vi "Calc_Vres.vi"(10 "S_Data in":dbl, 11 "P_Data in":dbl) -> (1 "Vres_FD":i32, 2 "Vres":dbl, 3 "Angle out":dbl)   [LabVIEW 2020]
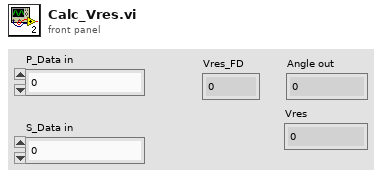
[diagram p1: front panel]
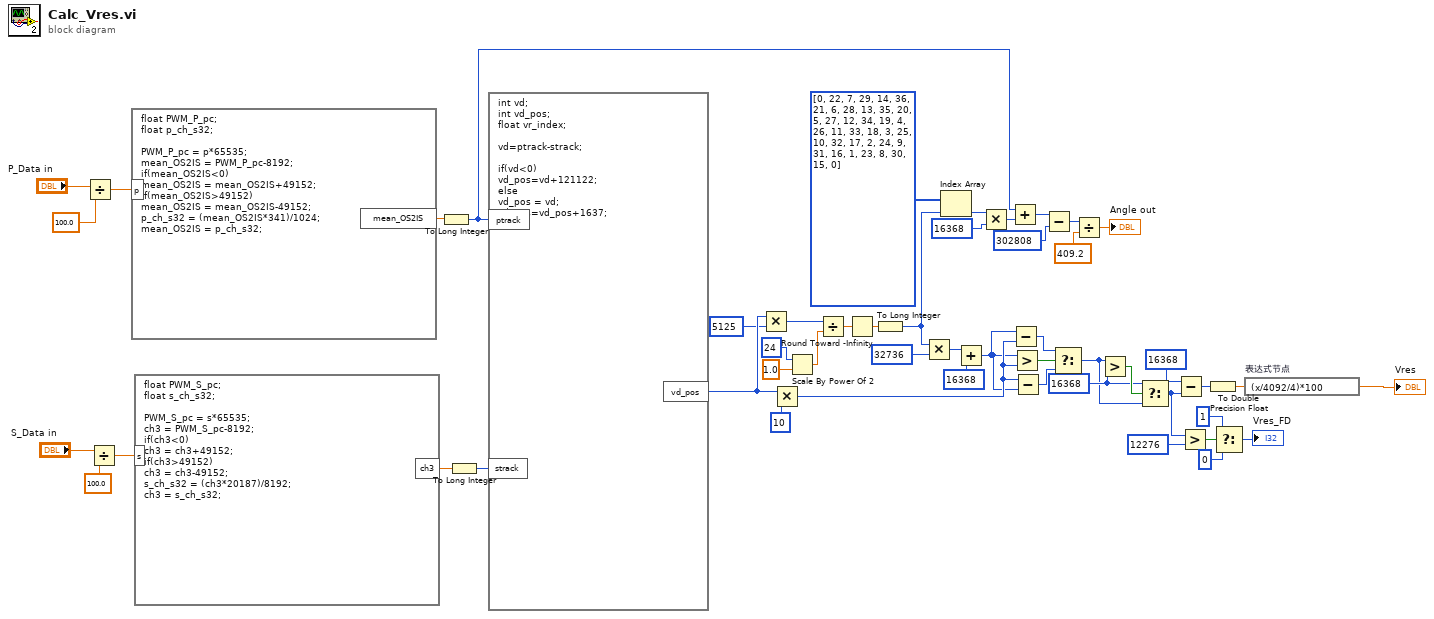
[diagram p0: block diagram]
diagram:
  w25 = 16368 ("y")
  n1 = Divide(x="P_Data in", y=100.0) -> (x/y=w12:dbl)
  n2 = Divide(x="S_Data in", y=100.0) -> (x/y=w10:dbl)
  n3 = formula code="float PWM_P_pc;\nfloat p_ch_s32;\n\nPWM_P_pc = p*65535;\nmean_OS2IS = PWM_P_pc-8192;\nif(mean_OS2IS<0)\nmean_OS2IS = mean_OS2IS+49152;\nif(mean_OS2IS>49152)\nmean_OS2IS = mean_OS2IS-49152;\np_ch_s32 = (mean_OS2IS*341)/1024;\nmean_OS2IS = p_ch_s32;"("p"=w12) -> ("mean_OS2IS"=w49:dbl)
  n4 = formula code="float PWM_S_pc;\nfloat s_ch_s32;\n\nPWM_S_pc = s*65535;\nch3 = PWM_S_pc-8192;\nif(ch3<0)\nch3 = ch3+49152;\nif(ch3>49152)\nch3 = ch3-49152;\ns_ch_s32 = (ch3*20187)/8192;\nch3 = s_ch_s32;"("s"=w10) -> ("ch3"=w50:dbl)
  n5 = To Long Integer(number=w49) -> (32bit integer=w42:i32)
  n6 = To Long Integer(number=w50) -> (32bit integer=w48:i32)
  n7 = formula code="int vd;\nint vd_pos;\nfloat vr_index;\n\nvd=ptrack-strack;\n\nif(vd<0)\nvd_pos=vd+121122;\nelse\nvd_pos = vd;\nvd_pos=vd_pos+1637;"("ptrack"=w42, "strack"=w48) -> ("vd_pos"=w17:i32)
  n8 = Multiply(x=w17, y=5125) -> (x*y=w15:i32)
  n9 = Multiply(x=w17, y=10) -> (x*y=w30:i32)
  n10 = Scale By Power Of 2(n=i16 24, x=1.0) -> (x*2^n=w14:dbl)
  n11 = Divide(x=w15, y=w14) -> (x/y=w13:dbl)
  n12 = Round Toward -Infinity(1:w13) -> (0:w47:dbl)
  n13 = To Long Integer(number=w47) -> (32bit integer=w36:i32)
  n14 = Multiply(x=w36, y=32736) -> (x*y=w34:i32)
  n15 = Index Array(array=i32[] [0, 22, 7, 29, 14, 36, 21, 6, 28, 13, 35, 20, 5, 27, 12, 34, 19, 4, 26, 11, 33, 18, 3, 25, 10, 32, 17, 2, 24, 9, 31, 16, 1, 23, 8, 30, 15, 0], index=w36) -> (element=w45:i32)
  n16 = Add(x=w34, y=16368) -> (x+y=w29:i32)
  n17 = Multiply(x=w45, y=16368) -> (x*y=w43:i32)
  n18 = Add(x=w42, y=w43) -> (x+y=w41:i32)
  n19 = Subtract(x=w29, y=w30) -> (x-y=w27:i32)
  n20 = Greater?(x=w29, y=w30) -> (0:w28:bool)
  n21 = Subtract(x=w30, y=w29) -> (x-y=w31:i32)
  n22 = Subtract(x=w41, y=302808) -> (x-y=w39:i32)
  n23 = Select(t=w27, s=w28, f=w31) -> (s? t:f=w24:i32)
  n24 = Divide(x=w39, y=409.2) -> (x/y=→"Angle out":dbl)
  n25 = Greater?(x=w24, y=w25) -> (0:w26:bool)
  n26 = Select(t=w25, s=w26, f=w24) -> (s? t:f=w8:i32)
  n27 = Subtract(x=16368 ("y"), y=w8) -> (x-y=w22:i32)
  n28 = Greater?(x=w8, y=12276) -> (0:w6:bool)
  n29 = To Double Precision Float(number=w22) -> (double precision float=w21:dbl)
  n30 = Select(t=1 ("y"), s=w6, f=0 ("y")) -> (s? t:f=→"Vres_FD":i32)
  n31 = expression code="(x/4092/4)*100" "表达式节点"(w21) -> (→"Vres":dbl)
